vi "R(T) T(t) SETP(t) with ramp332 DC ramp current(File overwrite Fixed)_1.vi"(0 "I":dbl=1e-06 min=1e-09 max=1.0 step=1e-06 format="%.4e", 1 "Ti":dbl min=0.0 max=400.0 format="%.3f", 2 "Tf":dbl=4.0 min=0.0 max=400.0 format="%.3f", 3 "Ramp":ext format="%.3f", 4 "Range":dbl=3.0 format="%.2f", 7 "Measurement":bool=TRUE, 8 "Auto\nTemp?":bool=TRUE) -> ()   [LabVIEW 2013]
panel:
  in  "Path":path
  in  "File name":string
  out "XY Graph":cluster{"X":dbl, "Y":dbl}[](graph)
  in  "Autorange":bool=TRUE
  in  "Volt Delay":u32=50
  in  "Voltmeter PLC":dbl=1.0 min=0.01 max=60.0 step=0.01 format="%.2f"
  in  "Voltage Compliance":dbl=12.0 min=0.1 max=105.0 step=0.1 format="%.2f"
  in  "minutes to wait before start":u32=5
  out "R/Ohm":dbl=1e-09 min=-1.0 step=1e-09 format="%.3e"
  out "T/K":dbl min=0.0 step=0.01 format="%.3f"
  out "?":cluster{dbl, dbl}[](graph)
  in  "Delay time":sgl min=0 step=1 format="%.2f"
  # "ON"
  # "OFF"
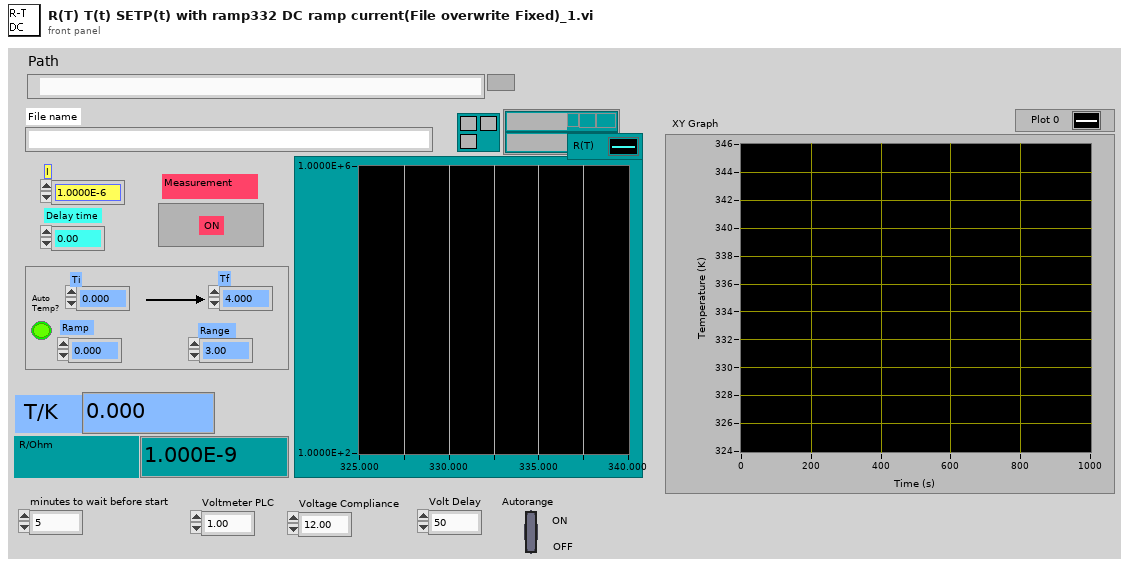
[diagram p1: front panel]
types:
  T1 = enum16{"open", "replace", "create", "open or create", "replace or create", "replace or create with confirmation"}
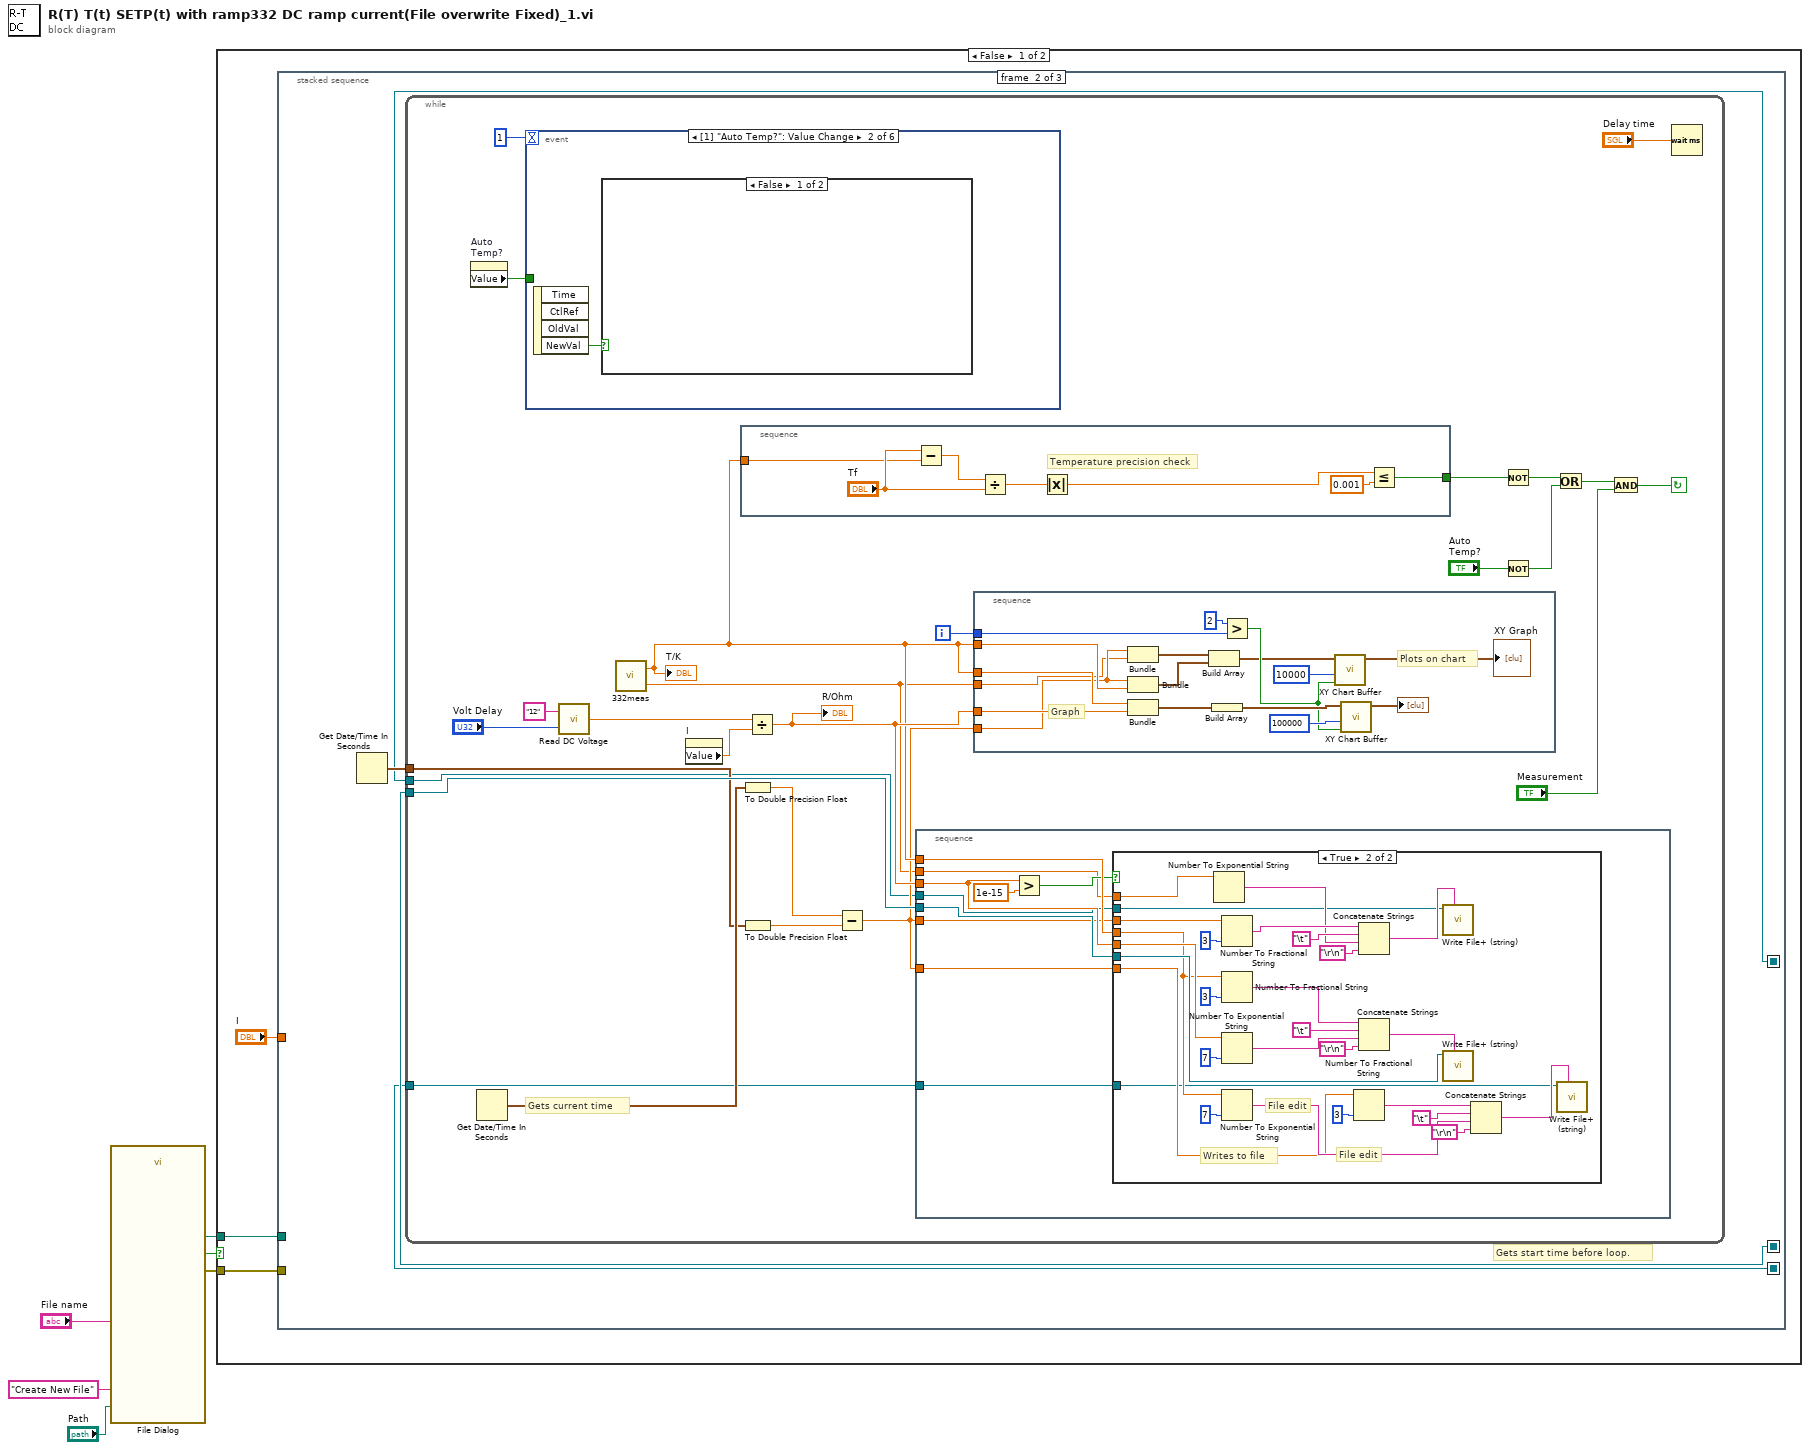
[diagram p0: block diagram]
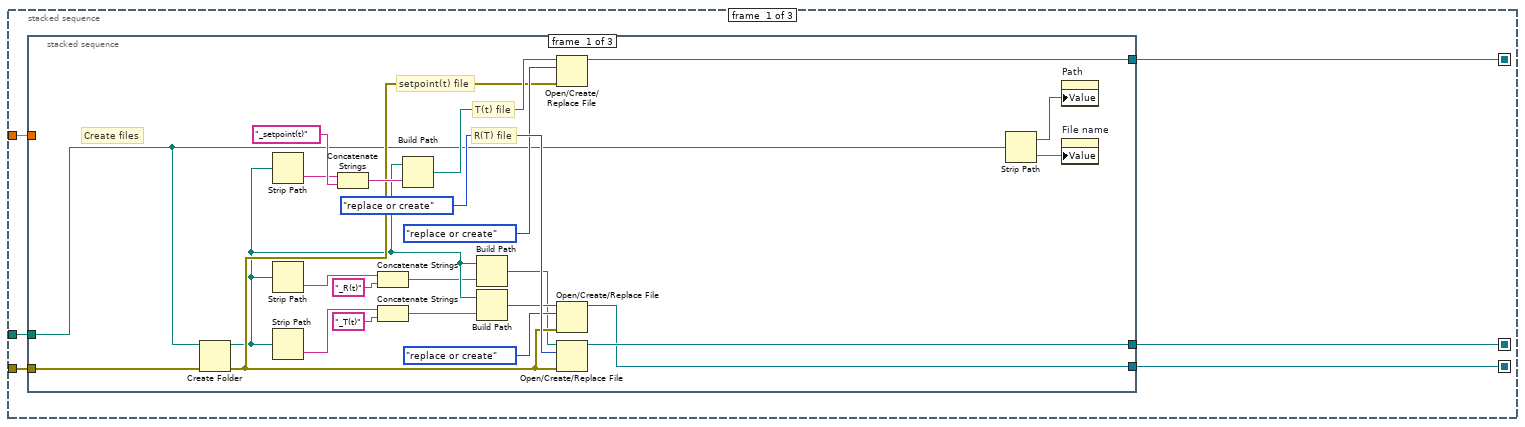
[diagram p2: hidden frame]
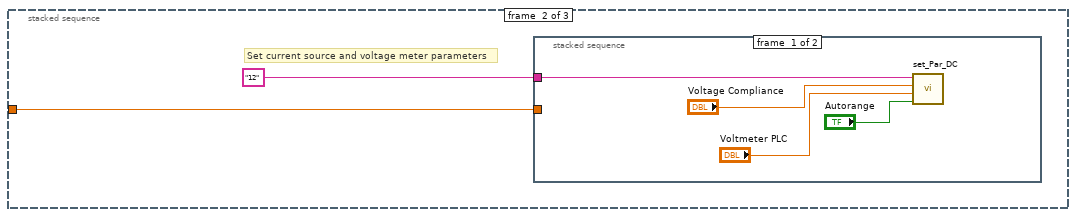
[diagram p3: hidden frame]
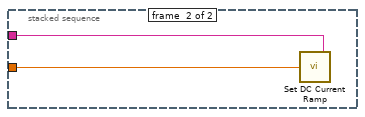
[diagram p4: hidden frame]
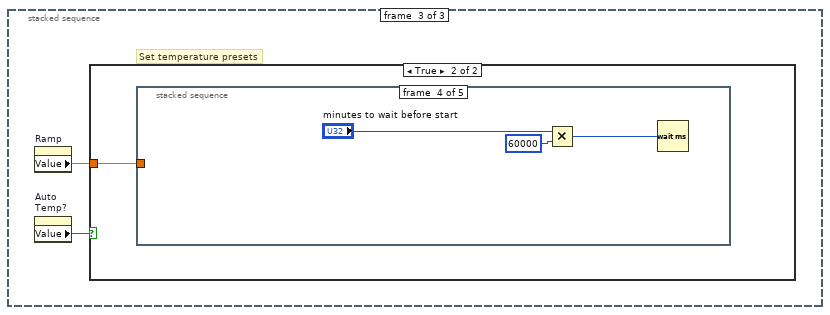
[diagram p5: hidden frame]
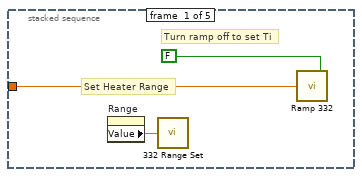
[diagram p7: hidden frame]
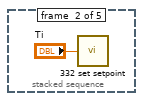
[diagram p8: hidden frame]
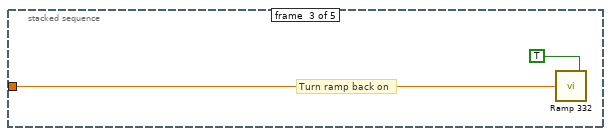
[diagram p9: hidden frame]
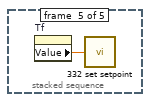
[diagram p10: hidden frame]
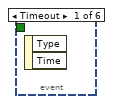
[diagram p12: hidden frame]
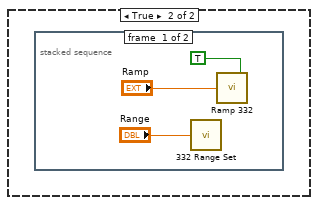
[diagram p13: hidden frame]
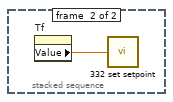
[diagram p14: hidden frame]
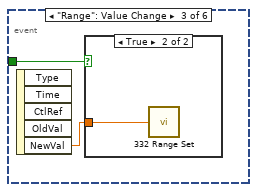
[diagram p15: hidden frame]
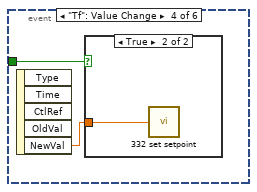
[diagram p17: hidden frame]
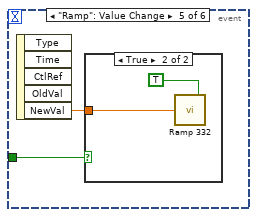
[diagram p19: hidden frame]
diagram:
  n1 = call "File Dialog"("start path"="Path", "prompt"="Create New File", "default name"="File name") -> ("selected path"=w3:path, "cancelled"=w1:bool, "error out"=w2:errorcluster)  [unwired: 9 in, 1 out]
  n2 = case shown="False" w1 {
    tunnel: w3 -> [w9 _]
    tunnel: w2 -> [w8 _]
    frame False {
      n3 = stacked-sequence {
        seq-local: [w15 _ _] -> [_ w64 w176]
        seq-local: [w13 _ _] -> [_ w62 w172]
        seq-local: [w12 _ _] -> [_ w61 _]
        tunnel: "I" -> [w14 _ w173]
        tunnel: w9 -> [w11 _ _]
        tunnel: w8 -> [w10 _ _]
        frame #0 {
          n4 = stacked-sequence {
            tunnel: [w39 _ _] -> w15
            tunnel: w14 -> [_ w40 _]
            tunnel: [w36 _ _] -> w13
            tunnel: [w26 _ _] -> w12
            tunnel: w11 -> [w19 _ _]
            tunnel: w10 -> [w18 _ _]
            frame #0 {
              # "setpoint(t) file"
              # "T(t) file"
              # "R(T) file"
              # "Create files"
              n5 = Create Folder(path (use dialog)=w19, error in=w18) -> (created path=w23:path, error out=w25:errorcluster)  [unwired: 1 in, 1 out]
              n6 = Strip Path(path=w23) -> (name=w28:string)  [unwired: 1 out]
              n7 = Strip Path(path=w23) -> (name=w21:string)  [unwired: 1 out]
              n8 = Strip Path(path=w23) -> (name=w35:string)  [unwired: 1 out]
              n9 = Concatenate Strings(w28, "_setpoint(t)" ("name or relative path")) -> (w30:string)
              n10 = Concatenate Strings(w21, "_R(t)" ("name or relative path")) -> (w20:string)
              n11 = Concatenate Strings(w35, "_T(t)" ("name or relative path")) -> (w33:string)
              n12 = Build Path(base path=w23, name or relative path=w30) -> (appended path=w31:path)
              n13 = Build Path(base path=w23, name or relative path=w20) -> (appended path=w24:path)
              n14 = Build Path(base path=w23, name or relative path=w33) -> (appended path=w32:path)
              n15 = Open/Create/Replace File(file path (use dialog)=w31, error in=w25, operation (0:open)=T1."replace or create") -> (refnum out=w26:refnum<file>)  [unwired: 3 in, 2 out]
              n16 = Open/Create/Replace File(file path (use dialog)=w32, error in=w25, operation (0:open)=T1."replace or create") -> (refnum out=w36:refnum<file>)  [unwired: 3 in, 2 out]
              n17 = Open/Create/Replace File(file path (use dialog)=w24, error in=w25, operation (0:open)=T1."replace or create") -> (refnum out=w39:refnum<file>)  [unwired: 3 in, 2 out]
              n18 = Strip Path(path=w19) -> (stripped path=w16:path, name=w17:string)
              n19 = property on="Path" class="Path"("Value"=w16) -> ()  [unwired: 2 in, 2 out]
              n20 = property on="File name" class="Str"("Value"=w17) -> ()  [unwired: 2 in, 2 out]
            }
            frame #1 {
              # "Set current source and voltage meter parameters"
              n21 = stacked-sequence {
                tunnel: "12" ("Address") -> [w45 w47]
                tunnel: w40 -> [_ w46]
                frame #0 {
                  n22 = call "set_Par_DC.vi"("Autorange"="Autorange", "Voltmeter PLC"="Voltmeter PLC", "Voltage Compliance"="Voltage Compliance", "Address"=w45) -> ()
                }
                frame #1 {
                  n23 = call "Set DC Current Ramp.vi"("Address"=w47, "Current"=w46) -> ()
                }
              }
            }
            frame #2 {
              # "Set temperature presets"
              n24 = property on="Ramp" class="DigNum (strict)"() -> ("Value"=w48:ext)  [unwired: 2 in, 2 out]
              n25 = property on="Auto\nTemp?" class="Bool (strict)"() -> ("Value"=w49:bool)  [unwired: 2 in, 2 out]
              n26 = case shown="True" w49 {
                tunnel: w48 -> [_ w50]
                frame False {
                }
                frame True {
                  n27 = stacked-sequence {
                    tunnel: w50 -> [w52 _ w56 _ _]
                    frame #0 {
                      # "Set Heater Range"
                      # "Turn ramp off to set Ti"
                      n28 = property on="Range" class="DigNum (strict)"() -> ("Value"=w51:dbl)  [unwired: 2 in, 2 out]
                      n29 = call "332 Range Set.vi"("Power Range: 93C\n0=OFF, 1=Low, 2=Med, 3=High"=w51) -> ()
                      n30 = call "Ramp 332.vi"("On"=FALSE, "K/min"=w52) -> ()
                    }
                    frame #1 {
                      n31 = call "332 set setpoint.vi"("Set Temperature SetPoint:332"="Ti") -> ()
                    }
                    frame #2 {
                      # "Turn ramp back on"
                      n32 = call "Ramp 332.vi"("On"=TRUE, "K/min"=w56) -> ()
                    }
                    frame #3 {
                      n33 = Multiply(x="minutes to wait before start", y=u32 60000) -> (x*y=w58:u32)
                      n34 = Wait (ms)(milliseconds to wait=w58) -> ()  [unwired: 1 out]
                    }
                    frame #4 {
                      n35 = property on="Tf" class="DigNum (strict)"() -> ("Value"=w60:dbl)  [unwired: 2 in, 2 out]
                      n36 = call "332 set setpoint.vi"("Set Temperature SetPoint:332"=w60) -> ()
                    }
                  }
                }
              }
            }
          }
        }
        frame #1 {
          # "Gets start time before loop."
          n37 = Get Date/Time In Seconds() -> (seconds since 1Jan1904=w63:timestamp)
          n38 = while {
            tunnel: w64 -> [w87]
            tunnel: w63 -> [w70]
            tunnel: w62 -> [w69]
            tunnel: w61 -> [w65]
            i -> [w90]
            stop <- w89 continue-if-true
            # "Gets current time"
            n39 = property on="Auto\nTemp?" class="Bool (strict)"() -> ("Value"=w83:bool)  [unwired: 2 in, 2 out]
            n40 = Get Date/Time In Seconds() -> (seconds since 1Jan1904=w72:timestamp)
            n41 = event shown="[1] \"Auto Temp?\": Value Change" {
              selector: _ -> [_ _ _ _ _ _]
              dyn-events: _ -> [_ _ _ _ _ _]
              timeout: 1 -> [_ _ _ _ _ _]
              tunnel: w83 -> [_ _ w159 w161 w164 _]
              event Timeout {
                n42 = event-data() -> ()  [unwired: 1 in, 2 out]
              }
              event "Auto\nTemp?": Value Change {
                n43 = event-data() -> ("NewVal"=w153:bool)  [unwired: 1 in, 3 out]
                n44 = case shown="False" w153 {
                  frame False {
                  }
                  frame True {
                    n45 = stacked-sequence {
                      frame #0 {
                        n46 = call "332 Range Set.vi"("Power Range: 93C\n0=OFF, 1=Low, 2=Med, 3=High"="Range") -> ()
                        n47 = call "Ramp 332.vi"("On"=TRUE, "K/min"="Ramp") -> ()
                      }
                      frame #1 {
                        n48 = property on="Tf" class="DigNum (strict)"() -> ("Value"=w157:dbl)  [unwired: 2 in, 2 out]
                        n49 = call "332 set setpoint.vi"("Set Temperature SetPoint:332"=w157) -> ()
                      }
                    }
                  }
                }
              }
              event "Range": Value Change {
                n50 = event-data() -> ("NewVal"=w158:dbl)  [unwired: 1 in, 4 out]
                n51 = case shown="True" w159 {
                  tunnel: w158 -> [_ w160]
                  frame False {
                  }
                  frame True {
                    n52 = call "332 Range Set.vi"("Power Range: 93C\n0=OFF, 1=Low, 2=Med, 3=High"=w160) -> ()
                  }
                }
              }
              event "Tf": Value Change {
                n53 = event-data() -> ("NewVal"=w162:dbl)  [unwired: 1 in, 4 out]
                n54 = case shown="True" w161 {
                  tunnel: w162 -> [_ w163]
                  frame False {
                  }
                  frame True {
                    n55 = call "332 set setpoint.vi"("Set Temperature SetPoint:332"=w163) -> ()
                  }
                }
              }
              event "Ramp": Value Change {
                n56 = event-data() -> ("NewVal"=w165:ext)  [unwired: 1 in, 4 out]
                n57 = case shown="True" w164 {
                  tunnel: w165 -> [_ w166]
                  frame False {
                  }
                  frame True {
                    n58 = call "Ramp 332.vi"("On"=TRUE, "K/min"=w166) -> ()
                  }
                }
              }
              event "I": Value Change {
                n59 = event-data() -> ("NewVal"=w168:dbl)  [unwired: 1 in, 4 out]
                n60 = stacked-sequence {
                  tunnel: w168 -> [_ w170]
                  frame #0 {
                    # "Wait until measurement\nfinished"
                    n61 = Wait (ms)(milliseconds to wait=u32 1000) -> ()  [unwired: 1 out]
                  }
                  frame #1 {
                    n62 = call "Set DC Current.vi"("Address"="24" ("address string"), "Current"=w170) -> ()
                  }
                }
              }
            }
            n63 = call "Read DC Voltage.vi"("Volt Delay"="Volt Delay", "Address"="12" ("address string")) -> ("Voltage"=w75:dbl)
            n64 = call "332meas.vi"() -> ("332 Temp [K]"=w68:dbl, "332 Temp Setpoint [K]"=w66:dbl)  [unwired: 1 in]
            "T/K" <- w68
            n65 = property on="I" class="DigNum (strict)"() -> ("Value"=w76:dbl)  [unwired: 2 in, 2 out]
            n66 = stacked-sequence {
              tunnel: [w146] -> w88
              tunnel: w68 -> [w147]
              frame #0 {
                # "Temperature precision check"
                n67 = Subtract(x="Tf", y=w147) -> (x-y=w150:dbl)
                n68 = Divide(x=w150, y="Tf") -> (x/y=w151:dbl)
                n69 = Absolute Value(x=w151) -> (abs(x)=w149:dbl)
                n70 = Less Or Equal?(x=w149, y=0.001) -> (x <= y?=w146:bool)
              }
            }
            n71 = To Double Precision Float(number=w72) -> (double precision float=w73:dbl)
            n72 = To Double Precision Float(number=w70) -> (double precision float=w71:dbl)
            n73 = Divide(x=w75, y=w76) -> (x/y=w78:dbl)
            "R/Ohm" <- w78
            n74 = Subtract(x=w73, y=w71) -> (x-y=w67:dbl)
            n75 = stacked-sequence {
              tunnel: w87 -> [w117]
              tunnel: w78 -> [w115]
              tunnel: w68 -> [w116]
              tunnel: w67 -> [w112]
              tunnel: w69 -> [w111]
              tunnel: w67 -> [w110]
              tunnel: w66 -> [w109]
              tunnel: w65 -> [w108]
              frame #0 {
                n76 = Greater?(x=w115, y=1e-15) -> (0:w114:bool)
                n77 = case shown="True" w114 {
                  tunnel: w117 -> [_ w142]
                  tunnel: w115 -> [_ w137]
                  tunnel: w116 -> [_ w129]
                  tunnel: w112 -> [_ w128]
                  tunnel: w111 -> [_ w127]
                  tunnel: w110 -> [_ w122]
                  tunnel: w109 -> [_ w120]
                  tunnel: w108 -> [_ w118]
                  frame False {
                  }
                  frame True {
                    # "Writes to file"
                    # "File edit"
                    # "File edit"
                    n78 = Number To Exponential String(number=w120) -> (E-format string=w119:string)  [unwired: 3 in]
                    n79 = Number To Fractional String(number=w122, precision (6)=3) -> (F-format string=w121:string)  [unwired: 2 in]
                    n80 = Number To Fractional String(number=w129, precision (6)=3) -> (F-format string=w145:string)  [unwired: 2 in]
                    n81 = Number To Exponential String(number=w137, precision (6)=7) -> (E-format string=w140:string)  [unwired: 2 in]
                    n82 = Number To Exponential String(number=w129, precision (6)=7) -> (E-format string=w132:string)  [unwired: 2 in]
                    n83 = Number To Fractional String(number=w128, precision (6)=3) -> (F-format string=w136:string)  [unwired: 2 in]
                    n84 = Concatenate Strings(w121, "\t", w119, "\r\n") -> (w124:string)
                    n85 = Concatenate Strings(w145, "\t", w140, "\r\n") -> (w144:string)
                    n86 = call <vilib>:"Write File+ (string).vi"("string"=w124, "refnum"=w118) -> ()  [unwired: 5 in, 3 out]
                    n87 = call <vilib>:"Write File+ (string).vi"("string"=w144, "refnum"=w142) -> ()  [unwired: 5 in, 3 out]
                    n88 = Concatenate Strings(w136, "\t", w132, "\r\n") -> (w135:string)
                    n89 = call <vilib>:"Write File+ (string).vi"("string"=w135, "refnum"=w127) -> ()  [unwired: 5 in, 3 out]
                  }
                }
              }
            }
            n90 = stacked-sequence {
              tunnel: w90 -> [w103]
              tunnel: w78 -> [w101]
              tunnel: w68 -> [w100]
              tunnel: w67 -> [w93]
              tunnel: w68 -> [w97]
              tunnel: w66 -> [w92]
              frame #0 {
                # "Plots on chart"
                # "Graph"
                n91 = Bundle(w93, "332 Temp Setpoint [K]"=w92) -> (w91:cluster{dbl, "332 Temp Setpoint [K]":dbl})  [unwired: 1 in]
                n92 = Bundle(w93, "332 Temp [K]"=w97) -> (w96:cluster{dbl, "332 Temp [K]":dbl})  [unwired: 1 in]
                n93 = Bundle("332 Temp [K]"=w100, w101) -> (w107:cluster{"332 Temp [K]":dbl, dbl})  [unwired: 1 in]
                n94 = Build Array(w91, w96) -> (w95:cluster{dbl, "332 Temp [K]":dbl}[])
                n95 = Build Array(w107) -> (w105:cluster{"332 Temp [K]":dbl, dbl}[])
                n96 = Greater?(x=2, y=w103) -> (0:w98:bool)
                n97 = call "XY Chart Buffer.vi"("clear first (no:F)"=w98, "chart length (points)"=10000, "new points"=w95) -> ("XY chart data"=→"XY Graph":cluster{"x":dbl, "y":dbl}[])  [unwired: 8 in]
                n98 = call "XY Chart Buffer.vi"("clear first (no:F)"=w98, "chart length (points)"=100000, "new points"=w105) -> ("XY chart data"=→"?":cluster{"x":dbl, "y":dbl}[])  [unwired: 8 in]
              }
            }
            n99 = Not(x=w88) -> (.not. x?=w85:bool)
            n100 = Not(x="Auto\nTemp?") -> (.not. x?=w79:bool)
            n101 = Or(x=w85, y=w79) -> (x .or. y?=w84:bool)
            n102 = And(x=w84, y="Measurement") -> (x .and. y?=w89:bool)
            n103 = Wait (ms)(milliseconds to wait="Delay time") -> ()  [unwired: 1 out]
          }
        }
        frame #2 {
          w174 = "12" ("Address")
          n104 = call "Send to Volt Meter.vi"("Address"=w174, "Data"=":trig:sour imm;:init") -> ()
          n105 = stacked-sequence {
            tunnel: w174 -> [w178 w179]
            tunnel: w173 -> [w177 _]
            frame #0 {
              n106 = call "Set DC Current Ramp to Zero.vi"("Address"=w178, "Current"=w177) -> ()
            }
            frame #1 {
              n107 = call "disarm.vi"("address string"=w179) -> ()  [unwired: 1 in, 1 out]
            }
          }
          n108 = Close File(refnum=w176) -> ()  [unwired: 1 in, 2 out]
          n109 = Close File(refnum=w172) -> ()  [unwired: 1 in, 2 out]
        }
      }
    }
    frame True {
    }
  }
